vi "example_02_convert.vi"() -> ()   [LabVIEW 2015, in "lv-unit-conversion.lvlib"] (continued)
"underlying_def"="", "description"=""}, {"symbol"="gal[US]/lbm", "name"="US gallon per pound-mass", "dimension"="L3/M", "is_si_unit"=TRUE, "category"="derived", "base_unit"="m3/kg", "conversion_reference"="DERIVED", "is_exact"=TRUE, "a"=0.0, "b"=0.003785411784, "c"=0.45359237, "d"=0.0, "underlying_def"="", "description"=""}, {"symbol"="gal[US]/sack[94lbm]", "name"="US gallon per 94-pound-sack", "dimension"="L3/M", "is_si_unit"=TRUE, "category"="derived", "base_unit"="m3/kg", "conversion_reference"="DERIVED", "is_exact"=TRUE, "a"=0.0, "b"=0.003785411784, "c"=42.63768278, "d"=0.0, "underlying_def"="", "description"=""}, {"symbol"="gal[US]/ton[UK]", "name"="US gallon per UK ton-mass", "dimension"="L3/M", "is_si_unit"=TRUE, "category"="derived", "base_unit"="m3/kg", "conversion_reference"="DERIVED", "is_exact"=TRUE, "a"=0.0, "b"=0.003785411784, "c"=1016.0469088, "d"=0.0, "underlying_def"="", "description"=""}, {"symbol"="gal[US]/ton[US]", "name"="US gallon per US ton-mass", "dimension"="L3/M", "is_si_unit"=TRUE, "category"="derived", "base_unit"="m3/kg", "conversion_reference"="DERIVED", "is_exact"=TRUE, "a"=0.0, "b"=0.003785411784, "c"=907.18474, "d"=0.0, "underlying_def"="", "description"=""}, {"symbol"="L/kg", "name"="litre per kilogram", "dimension"="L3/M", "is_si_unit"=TRUE, "category"="derived", "base_unit"="m3/kg", "conversion_reference"="DERIVED", "is_exact"=TRUE, "a"=0.0, "b"=0.001, "c"=1.0, "d"=0.0, "underlying_def"="", "description"=""}, {"symbol"="L/t", "name"="litre per tonne", "dimension"="L3/M", "is_si_unit"=TRUE, "category"="derived", "base_unit"="m3/kg", "conversion_reference"="DERIVED", "is_exact"=TRUE, "a"=0.0, "b"=1e-06, "c"=1.0, "d"=0.0, "underlying_def"="", "description"=""}, {"symbol"="L/ton[UK]", "name"="litre per UK ton-mass", "dimension"="L3/M", "is_si_unit"=TRUE, "category"="derived", "base_unit"="m3/kg", "conversion_reference"="DERIVED", "is_exact"=TRUE, "a"=0.0, "b"=0.001, "c"=1016.0469088, "d"=0.0, "underlying_def"="", "description"=""}, {"symbol"="m3/g", "name"="cubic metre per gram", "dimension"="L3/M", "is_si_unit"=TRUE, "category"="derived", "base_unit"="m3/kg", "conversion_reference"="DERIVED", "is_exact"=TRUE, "a"=0.0, "b"=1000.0, "c"=1.0, "d"=0.0, "underlying_def"="", "description"=""}, {"symbol"="m3/t", "name"="cubic metre per tonne", "dimension"="L3/M", "is_si_unit"=TRUE, "category"="derived", "base_unit"="m3/kg", "conversion_reference"="DERIVED", "is_exact"=TRUE, "a"=0.0, "b"=0.001, "c"=1.0, "d"=0.0, "underlying_def"="", "description"=""}, {"symbol"="m3/ton[UK]", "name"="cubic metre per UK ton-mass", "dimension"="L3/M", "is_si_unit"=TRUE, "category"="derived", "base_unit"="m3/kg", "conversion_reference"="DERIVED", "is_exact"=TRUE, "a"=0.0, "b"=1.0, "c"=1016.0469088, "d"=0.0, "underlying_def"="", "description"=""}, {"symbol"="m3/ton[US]", "name"="cubic metre per US ton-mass", "dimension"="L3/M", "is_si_unit"=TRUE, "category"="derived", "base_unit"="m3/kg", "conversion_reference"="DERIVED", "is_exact"=TRUE, "a"=0.0, "b"=1.0, "c"=907.18474, "d"=0.0, "underlying_def"="", "description"=""}, {"symbol"="m3/mol", "name"="cubic metre per gram-mole", "dimension"="L3/N", "is_si_unit"=TRUE, "category"="derived", "base_unit"="", "conversion_reference"="", "is_exact"=FALSE, "a"=0.0, "b"=0.0, "c"=0.0, "d"=0.0, "underlying_def"="", "description"=""}, {"symbol"="dm3/kmol", "name"="cubic decimetre per kilogram-mole", "dimension"="L3/N", "is_si_unit"=TRUE, "category"="derived", "base_unit"="m3/mol", "conversion_reference"="DERIVED", "is_exact"=TRUE, "a"=0.0, "b"=1e-06, "c"=1.0, "d"=0.0, "underlying_def"="", "description"=""}, {"symbol"="ft3/lbmol", "name"="cubic foot per pound-mass-mole", "dimension"="L3/N", "is_si_unit"=TRUE, "category"="derived", "base_unit"="m3/mol", "conversion_reference"="DERIVED", "is_exact"=TRUE, "a"=0.0, "b"=0.028316846592, "c"=453.59237, "d"=0.0, "underlying_def"="", "description"=""}, {"symbol"="L/kmol", "name"="litre per kilogram-mole", "dimension"="L3/N", "is_si_unit"=TRUE, "category"="derived", "base_unit"="m3/mol", "conversion_reference"="DERIVED", "is_exact"=TRUE, "a"=0.0, "b"=1e-06, "c"=1.0, "d"=0.0, "underlying_def"="", "description"=""}, {"symbol"="L/mol", "name"="litre per gram-mole", "dimension"="L3/N", "is_si_unit"=TRUE, "category"="derived", "base_unit"="m3/mol", "conversion_reference"="DERIVED", "is_exact"=TRUE, "a"=0.0, "b"=0.001, "c"=1.0, "d"=0.0, "underlying_def"="", "description"=""}, {"symbol"="m3/kmol", "name"="cubic metre per kilogram-mole", "dimension"="L3/N", "is_si_unit"=TRUE, "category"="derived", "base_unit"="m3/mol", "conversion_reference"="DERIVED", "is_exact"=TRUE, "a"=0.0, "b"=0.001, "c"=1.0, "d"=0.0, "underlying_def"="", "description"=""}, {"symbol"="m3/s", "name"="cubic metre per second", "dimension"="L3/T", "is_si_unit"=TRUE, "category"="derived", "base_unit"="", "conversion_reference"="", "is_exact"=FALSE, "a"=0.0, "b"=0.0, "c"=0.0, "d"=0.0, "underlying_def"="", "description"=""}, {"symbol"="1/30 cm3/min", "name"="cubic centimetre per thirty minute", "dimension"="L3/T", "is_si_unit"=TRUE, "category"="derived", "base_unit"="m3/s", "conversion_reference"="DERIVED", "is_exact"=TRUE, "a"=0.0, "b"=1e-06, "c"=1800.0, "d"=0.0, "underlying_def"="", "description"=""}, {"symbol"="1000 bbl/d", "name"="thousand barrel per day", "dimension"="L3/T", "is_si_unit"=TRUE, "category"="derived", "base_unit"="m3/s", "conversion_reference"="DERIVED", "is_exact"=TRUE, "a"=0.0, "b"=158.987294928, "c"=86400.0, "d"=0.0, "underlying_def"="", "description"=""}, {"symbol"="1000 ft3/d", "name"="thousand cubic foot per day", "dimension"="L3/T", "is_si_unit"=TRUE, "category"="derived", "base_unit"="m3/s", "conversion_reference"="DERIVED", "is_exact"=TRUE, "a"=0.0, "b"=28.316846592, "c"=86400.0, "d"=0.0, "underlying_def"="", "description"=""}, {"symbol"="1000 m3/d", "name"="thousand cubic metre per day", "dimension"="L3/T", "is_si_unit"=TRUE, "category"="derived", "base_unit"="m3/s", "conversion_reference"="DERIVED", "is_exact"=TRUE, "a"=0.0, "b"=1000.0, "c"=86400.0, "d"=0.0, "underlying_def"="", "description"=""}, {"symbol"="1000 m3/h", "name"="thousand cubic metre per hour", "dimension"="L3/T", "is_si_unit"=TRUE, "category"="derived", "base_unit"="m3/s", "conversion_reference"="DERIVED", "is_exact"=TRUE, "a"=0.0, "b"=1000.0, "c"=3600.0, "d"=0.0, "underlying_def"="", "description"=""}, {"symbol"="1E6 bbl/d", "name"="million barrel per day", "dimension"="L3/T", "is_si_unit"=TRUE, "category"="derived", "base_unit"="m3/s", "conversion_reference"="DERIVED", "is_exact"=TRUE, "a"=0.0, "b"=158987.294928, "c"=86400.0, "d"=0.0, "underlying_def"="", "description"=""}, {"symbol"="1E6 ft3/d", "name"="million cubic foot per day", "dimension"="L3/T", "is_si_unit"=TRUE, "category"="derived", "base_unit"="m3/s", "conversion_reference"="DERIVED", "is_exact"=TRUE, "a"=0.0, "b"=28316.846592, "c"=86400.0, "d"=0.0, "underlying_def"="", "description"=""}, {"symbol"="1E6 m3/d", "name"="million cubic metre per day", "dimension"="L3/T", "is_si_unit"=TRUE, "category"="derived", "base_unit"="m3/s", "conversion_reference"="DERIVED", "is_exact"=TRUE, "a"=0.0, "b"=1000000.0, "c"=86400.0, "d"=0.0, "underlying_def"="", "description"=""}, {"symbol"="bbl/d", "name"="barrel per day", "dimension"="L3/T", "is_si_unit"=TRUE, "category"="derived", "base_unit"="m3/s", "conversion_reference"="DERIVED", "is_exact"=TRUE, "a"=0.0, "b"=0.158987294928, "c"=86400.0, "d"=0.0, "underlying_def"="", "description"=""}, {"symbol"="bbl/h", "name"="barrel per hour", "dimension"="L3/T", "is_si_unit"=TRUE, "category"="derived", "base_unit"="m3/s", "conversion_reference"="DERIVED", "is_exact"=TRUE, "a"=0.0, "b"=0.158987294928, "c"=3600.0, "d"=0.0, "underlying_def"="", "description"=""}, {"symbol"="bbl/min", "name"="barrel per minute", "dimension"="L3/T", "is_si_unit"=TRUE, "category"="derived", "base_unit"="m3/s", "conversion_reference"="DERIVED", "is_exact"=TRUE, "a"=0.0, "b"=0.158987294928, "c"=60.0, "d"=0.0, "underlying_def"="", "description"=""}, {"symbol"="cm3/h", "name"="cubic centimetre per hour", "dimension"="L3/T", "is_si_unit"=TRUE, "category"="derived", "base_unit"="m3/s", "conversion_reference"="DERIVED", "is_exact"=TRUE, "a"=0.0, "b"=1e-06, "c"=3600.0, "d"=0.0, "underlying_def"="", "description"=""}, {"symbol"="cm3/min", "name"="cubic centimetre per minute", "dimension"="L3/T", "is_si_unit"=TRUE, "category"="derived", "base_unit"="m3/s", "conversion_reference"="DERIVED", "is_exact"=TRUE, "a"=0.0, "b"=1e-06, "c"=60.0, "d"=0.0, "underlying_def"="", "description"=""}, {"symbol"="cm3/s", "name"="cubic centimetre per second", "dimension"="L3/T", "is_si_unit"=TRUE, "category"="derived", "base_unit"="m3/s", "conversion_reference"="DERIVED", "is_exact"=TRUE, "a"=0.0, "b"=1e-06, "c"=1.0, "d"=0.0, "underlying_def"="", "description"=""}, {"symbol"="dm3/s", "name"="cubic decimetre per second", "dimension"="L3/T", "is_si_unit"=TRUE, "category"="derived", "base_unit"="m3/s", "conversion_reference"="DERIVED", "is_exact"=TRUE, "a"=0.0, "b"=0.001, "c"=1.0, "d"=0.0, "underlying_def"="", "description"=""}, {"symbol"="ft3/d", "name"="cubic foot per day", "dimension"="L3/T", "is_si_unit"=TRUE, "category"="derived", "base_unit"="m3/s", "conversion_reference"="DERIVED", "is_exact"=TRUE, "a"=0.0, "b"=0.028316846592, "c"=86400.0, "d"=0.0, "underlying_def"="", "description"=""}, {"symbol"="ft3/h", "name"="cubic foot per hour", "dimension"="L3/T", "is_si_unit"=TRUE, "category"="derived", "base_unit"="m3/s", "conversion_reference"="DERIVED", "is_exact"=TRUE, "a"=0.0, "b"=0.028316846592, "c"=3600.0, "d"=0.0, "underlying_def"="", "description"=""}, {"symbol"="ft3/min", "name"="cubic foot per minute", "dimension"="L3/T", "is_si_unit"=TRUE, "category"="derived", "base_unit"="m3/s", "conversion_reference"="DERIVED", "is_exact"=TRUE, "a"=0.0, "b"=0.028316846592, "c"=60.0, "d"=0.0, "underlying_def"="", "description"=""}, {"symbol"="ft3/s", "name"="cubic foot per second", "dimension"="L3/T", "is_si_unit"=TRUE, "category"="derived", "base_unit"="m3/s", "conversion_reference"="DERIVED", "is_exact"=TRUE, "a"=0.0, "b"=0.028316846592, "c"=1.0, "d"=0.0, "underlying_def"="", "description"=""}, {"symbol"="gal[UK]/d", "name"="UK gallon per day", "dimension"="L3/T", "is_si_unit"=TRUE, "category"="derived", "base_unit"="m3/s", "conversion_reference"="DERIVED", "is_exact"=TRUE, "a"=0.0, "b"=0.00454609, "c"=86400.0, "d"=0.0, "underlying_def"="", "description"=""}, {"symbol"="gal[UK]/h", "name"="UK gallon per hour", "dimension"="L3/T", "is_si_unit"=TRUE, "category"="derived", "base_unit"="m3/s", "conversion_reference"="DERIVED", "is_exact"=TRUE, "a"=0.0, "b"=0.00454609, "c"=3600.0, "d"=0.0, "underlying_def"="", "description"=""}, {"symbol"="gal[UK]/min", "name"="UK gallon per minute", "dimension"="L3/T", "is_si_unit"=TRUE, "category"="derived", "base_unit"="m3/s", "conversion_reference"="DERIVED", "is_exact"=TRUE, "a"=0.0, "b"=0.00454609, "c"=60.0, "d"=0.0, "underlying_def"="", "description"=""}, {"symbol"="gal[US]/d", "name"="US gallon per day", "dimension"="L3/T", "is_si_unit"=TRUE, "category"="derived", "base_unit"="m3/s", "conversion_reference"="DERIVED", "is_exact"=TRUE, "a"=0.0, "b"=0.003785411784, "c"=86400.0, "d"=0.0, "underlying_def"="", "description"=""}, {"symbol"="gal[US]/h", "name"="US gallon per hour", "dimension"="L3/T", "is_si_unit"=TRUE, "category"="derived", "base_unit"="m3/s", "conversion_reference"="DERIVED", "is_exact"=TRUE, "a"=0.0, "b"=0.003785411784, "c"=3600.0, "d"=0.0, "underlying_def"="", "description"=""}, {"symbol"="gal[US]/min", "name"="US gallon per minute", "dimension"="L3/T", "is_si_unit"=TRUE, "category"="derived", "base_unit"="m3/s", "conversion_reference"="DERIVED", "is_exact"=TRUE, "a"=0.0, "b"=0.003785411784, "c"=60.0, "d"=0.0, "underlying_def"="", "description"=""}, {"symbol"="L/h", "name"="litre per hour", "dimension"="L3/T", "is_si_unit"=TRUE, "category"="derived", "base_unit"="m3/s", "conversion_reference"="DERIVED", "is_exact"=TRUE, "a"=0.0, "b"=0.001, "c"=3600.0, "d"=0.0, "underlying_def"="", "description"=""}, {"symbol"="L/min", "name"="litre per minute", "dimension"="L3/T", "is_si_unit"=TRUE, "category"="derived", "base_unit"="m3/s", "conversion_reference"="DERIVED", "is_exact"=TRUE, "a"=0.0, "b"=0.001, "c"=60.0, "d"=0.0, "underlying_def"="", "description"=""}, {"symbol"="L/s", "name"="litre per second", "dimension"="L3/T", "is_si_unit"=TRUE, "category"="derived", "base_unit"="m3/s", "conversion_reference"="DERIVED", "is_exact"=TRUE, "a"=0.0, "b"=0.001, "c"=1.0, "d"=0.0, "underlying_def"="", "description"=""}, {"symbol"="m3/d", "name"="cubic metre per day", "dimension"="L3/T", "is_si_unit"=TRUE, "category"="derived", "base_unit"="m3/s", "conversion_reference"="DERIVED", "is_exact"=TRUE, "a"=0.0, "b"=1.0, "c"=86400.0, "d"=0.0, "underlying_def"="", "description"=""}, {"symbol"="m3/h", "name"="cubic metre per hour", "dimension"="L3/T", "is_si_unit"=TRUE, "category"="derived", "base_unit"="m3/s", "conversion_reference"="DERIVED", "is_exact"=TRUE, "a"=0.0, "b"=1.0, "c"=3600.0, "d"=0.0, "underlying_def"="", "description"=""}, {"symbol"="m3/min", "name"="cubic metre per minute", "dimension"="L3/T", "is_si_unit"=TRUE, "category"="derived", "base_unit"="m3/s", "conversion_reference"="DERIVED", "is_exact"=TRUE, "a"=0.0, "b"=1.0, "c"=60.0, "d"=0.0, "underlying_def"="", "description"=""}, {"symbol"="m3/s2", "name"="cubic metre per second squared", "dimension"="L3/T2", "is_si_unit"=TRUE, "category"="derived", "base_unit"="", "conversion_reference"="", "is_exact"=FALSE, "a"=0.0, "b"=0.0, "c"=0.0, "d"=0.0, "underlying_def"="", "description"=""}, {"symbol"="bbl/d2", "name"="(barrel per day) per day", "dimension"="L3/T2", "is_si_unit"=TRUE, "category"="derived", "base_unit"="m3/s2", "conversion_reference"="DERIVED", "is_exact"=TRUE, "a"=0.0, "b"=0.158987294928, "c"=7464960000.0, "d"=0.0, "underlying_def"="", "description"=""}, {"symbol"="bbl/h2", "name"="(barrel per hour) per hour", "dimension"="L3/T2", "is_si_unit"=TRUE, "category"="derived", "base_unit"="m3/s2", "conversion_reference"="DERIVED", "is_exact"=TRUE, "a"=0.0, "b"=0.158987294928, "c"=12960000.0, "d"=0.0, "underlying_def"="", "description"=""}, {"symbol"="dm3/s2", "name"="(cubic decimetre per second) per second", "dimension"="L3/T2", "is_si_unit"=TRUE, "category"="derived", "base_unit"="m3/s2", "conversion_reference"="DERIVED", "is_exact"=TRUE, "a"=0.0, "b"=0.001, "c"=1.0, "d"=0.0, "underlying_def"="", "description"=""}, {"symbol"="ft3/d2", "name"="(cubic foot per day) per day", "dimension"="L3/T2", "is_si_unit"=TRUE, "category"="derived", "base_unit"="m3/s2", "conversion_reference"="DERIVED", "is_exact"=TRUE, "a"=0.0, "b"=0.028316846592, "c"=7464960000.0, "d"=0.0, "underlying_def"="", "description"=""}, {"symbol"="ft3/h2", "name"="(cubic foot per hour) per hour", "dimension"="L3/T2", "is_si_unit"=TRUE, "category"="derived", "base_unit"="m3/s2", "conversion_reference"="DERIVED", "is_exact"=TRUE, "a"=0.0, "b"=0.028316846592, "c"=12960000.0, "d"=0.0, "underlying_def"="", "description"=""}, {"symbol"="ft3/min2", "name"="(cubic foot per minute) per minute", "dimension"="L3/T2", "is_si_unit"=TRUE, "category"="derived", "base_unit"="m3/s2", "conversion_reference"="DERIVED", "is_exact"=TRUE, "a"=0.0, "b"=0.028316846592, "c"=3600.0, "d"=0.0, "underlying_def"="", "description"=""}, {"symbol"="ft3/s2", "name"="(cubic foot per second) per second", "dimension"="L3/T2", "is_si_unit"=TRUE, "category"="derived", "base_unit"="m3/s2", "conversion_reference"="DERIVED", "is_exact"=TRUE, "a"=0.0, "b"=0.028316846592, "c"=1.0, "d"=0.0, "underlying_def"="", "description"=""}, {"symbol"="gal[UK]/h2", "name"="(UK gallon per hour) per hour", "dimension"="L3/T2", "is_si_unit"=TRUE, "category"="derived", "base_unit"="m3/s2", "conversion_reference"="DERIVED", "is_exact"=TRUE, "a"=0.0, "b"=0.00454609, "c"=12960000.0, "d"=0.0, "underlying_def"="", "description"=""}, {"symbol"="gal[UK]/min2", "name"="(UK gallon per minute) per minute", "dimension"="L3/T2", "is_si_unit"=TRUE, "category"="derived", "base_unit"="m3/s2", "conversion_reference"="DERIVED", "is_exact"=TRUE, "a"=0.0, "b"=0.00454609, "c"=3600.0, "d"=0.0, "underlying_def"="", "description"=""}, {"symbol"="gal[US]/h2", "name"="(US gallon per hour) per hour", "dimension"="L3/T2", "is_si_unit"=TRUE, "category"="derived", "base_unit"="m3/s2", "conversion_reference"="DERIVED", "is_exact"=TRUE, "a"=0.0, "b"=0.003785411784, "c"=12960000.0, "d"=0.0, "underlying_def"="", "description"=""}, {"symbol"="gal[US]/min2", "name"="(US gallon per minute) per minute", "dimension"="L3/T2", "is_si_unit"=TRUE, "category"="derived", "base_unit"="m3/s2", "conversion_reference"="DERIVED", "is_exact"=TRUE, "a"=0.0, "b"=0.003785411784, "c"=3600.0, "d"=0.0, "underlying_def"="", "description"=""}, {"symbol"="L/s2", "name"="(litre per second) per second", "dimension"="L3/T2", "is_si_unit"=TRUE, "category"="derived", "base_unit"="m3/s2", "conversion_reference"="DERIVED", "is_exact"=TRUE, "a"=0.0, "b"=0.001, "c"=1.0, "d"=0.0, "underlying_def"="", "description"=""}, {"symbol"="m3/d2", "name"="(cubic metre per day) per day", "dimension"="L3/T2", "is_si_unit"=TRUE, "category"="derived", "base_unit"="m3/s2", "conversion_reference"="DERIVED", "is_exact"=TRUE, "a"=0.0, "b"=1.0, "c"=7464960000.0, "d"=0.0, "underlying_def"="", "description"=""}, {"symbol"="ohm.m", "name"="ohm metre", "dimension"="L3M/I2T3", "is_si_unit"=TRUE, "category"="derived", "base_unit"="", "conversion_reference"="", "is_exact"=FALSE, "a"=0.0, "b"=0.0, "c"=0.0, "d"=0.0, "underlying_def"="", "description"=""}, {"symbol"="kohm.m", "name"="kiloohm metre", "dimension"="L3M/I2T3", "is_si_unit"=TRUE, "category"="derived", "base_unit"="ohm.m", "conversion_reference"="DERIVED", "is_exact"=TRUE, "a"=0.0, "b"=1000.0, "c"=1.0, "d"=0.0, "underlying_def"="", "description"=""}, {"symbol"="nohm.mil2/ft", "name"="nanoohm square mil per foot", "dimension"="L3M/I2T3", "is_si_unit"=TRUE, "category"="derived", "base_unit"="ohm.m", "conversion_reference"="DERIVED", "is_exact"=TRUE, "a"=0.0, "b"=6.4516e-19, "c"=0.3048, "d"=0.0, "underlying_def"="", "description"=""}, {"symbol"="nohm.mm2/m", "name"="nanoohm square milimetre per metre", "dimension"="L3M/I2T3", "is_si_unit"=TRUE, "category"="derived", "base_unit"="ohm.m", "conversion_reference"="DERIVED", "is_exact"=TRUE, "a"=0.0, "b"=1e-15, "c"=1.0, "d"=0.0, "underlying_def"="", "description"=""}, {"symbol"="ohm.cm", "name"="ohm centimetre", "dimension"="L3M/I2T3", "is_si_unit"=TRUE, "category"="derived", "base_unit"="ohm.m", "conversion_reference"="DERIVED", "is_exact"=TRUE, "a"=0.0, "b"=0.01, "c"=1.0, "d"=0.0, "underlying_def"="", "description"=""}, {"symbol"="ohm.m2/m", "name"="ohm square metre per metre", "dimension"="L3M/I2T3", "is_si_unit"=TRUE, "category"="derived", "base_unit"="ohm.m", "conversion_reference"="DERIVED", "is_exact"=TRUE, "a"=0.0, "b"=1.0, "c"=1.0, "d"=0.0, "underlying_def"="", "description"=""}, {"symbol"="Wb.m", "name"="weber metre", "dimension"="L3M/IT2", "is_si_unit"=TRUE, "category"="derived", "base_unit"="", "conversion_reference"="", "is_exact"=FALSE, "a"=0.0, "b"=0.0, "c"=0.0, "d"=0.0, "underlying_def"="", "description"=""}, {"symbol"="N.m2", "name"="newton square metre", "dimension"="L3M/T2", "is_si_unit"=TRUE, "category"="derived", "base_unit"="", "conversion_reference"="", "is_exact"=FALSE, "a"=0.0, "b"=0.0, "c"=0.0, "d"=0.0, "underlying_def"="", "description"=""}, {"symbol"="dyne.cm2", "name"="dyne square centimetre", "dimension"="L3M/T2", "is_si_unit"=TRUE, "category"="derived", "base_unit"="N.m2", "conversion_reference"="DERIVED", "is_exact"=TRUE, "a"=0.0, "b"=1e-09, "c"=1.0, "d"=0.0, "underlying_def"="", "description"=""}, {"symbol"="kgf.m2", "name"="thousand gram-force square metre", "dimension"="L3M/T2", "is_si_unit"=TRUE, "category"="derived", "base_unit"="N.m2", "conversion_reference"="DERIVED", "is_exact"=TRUE, "a"=0.0, "b"=9.80665, "c"=1.0, "d"=0.0, "underlying_def"="", "description"=""}, {"symbol"="kN.m2", "name"="kilonewton square metre", "dimension"="L3M/T2", "is_si_unit"=TRUE, "category"="derived", "base_unit"="N.m2", "conversion_reference"="DERIVED", "is_exact"=TRUE, "a"=0.0, "b"=1000.0, "c"=1.0, "d"=0.0, "underlying_def"="", "description"=""}, {"symbol"="lbf.in2", "name"="pound-force square inch", "dimension"="L3M/T2", "is_si_unit"=TRUE, "category"="derived", "base_unit"="N.m2", "conversion_reference"="DERIVED", "is_exact"=TRUE, "a"=0.0, "b"=0.002869814657301464, "c"=1.0, "d"=0.0, "underlying_def"="", "description"=""}, {"symbol"="mN.m2", "name"="millinewton square metre", "dimension"="L3M/T2", "is_si_unit"=TRUE, "category"="derived", "base_unit"="N.m2", "conversion_reference"="DERIVED", "is_exact"=TRUE, "a"=0.0, "b"=0.001, "c"=1.0, "d"=0.0, "underlying_def"="", "description"=""}, {"symbol"="pdl.cm2", "name"="poundal square centimetre", "dimension"="L3M/T2", "is_si_unit"=TRUE, "category"="derived", "base_unit"="N.m2", "conversion_reference"="DERIVED", "is_exact"=TRUE, "a"=0.0, "b"=1.38254954376e-05, "c"=1.0, "d"=0.0, "underlying_def"="", "description"=""}, {"symbol"="tonf[UK].ft2", "name"="UK ton-force square foot", "dimension"="L3M/T2", "is_si_unit"=TRUE, "category"="derived", "base_unit"="N.m2", "conversion_reference"="DERIVED", "is_exact"=TRUE, "a"=0.0, "b"=925.6874158591603, "c"=1.0, "d"=0.0, "underlying_def"="", "description"=""}, {"symbol"="tonf[US].ft2", "name"="US ton-force square foot", "dimension"="L3M/T2", "is_si_unit"=TRUE, "category"="derived", "base_unit"="N.m2", "conversion_reference"="DERIVED", "is_exact"=TRUE, "a"=0.0, "b"=826.5066213028217, "c"=1.0, "d"=0.0, "underlying_def"="", "description"=""}, {"symbol"="m2/(Pa.s)", "name"="square metre per pascal second", "dimension"="L3T/M", "is_si_unit"=TRUE, "category"="derived", "base_unit"="", "conversion_reference"="", "is_exact"=FALSE, "a"=0.0, "b"=0.0, "c"=0.0, "d"=0.0, "underlying_def"="", "description"=""}, {"symbol"="TD[API]/(Pa.s)", "name"="teradarcy-API per pascal second", "dimension"="L3T/M", "is_si_unit"=TRUE, "category"="derived", "base_unit"="", "conversion_reference"="", "is_exact"=FALSE, "a"=0.0, "b"=0.0, "c"=0.0, "d"=0.0, "underlying_def"="m2/(Pa.s)", "description"=""}, {"symbol"="bbl/(ft.psi.d)", "name"="barrel per day foot psi", "dimension"="L3T/M", "is_si_unit"=TRUE, "category"="derived", "base_unit"="m2/(Pa.s)", "conversion_reference"="DERIVED", "is_exact"=TRUE, "a"=0.0, "b"=0.00010257224319574849, "c"=117142.67073583299, "d"=0.0, "underlying_def"="", "description"=""}, {"symbol"="ft3/(ft.psi.d)", "name"="cubic foot per day foot psi", "dimension"="L3T/M", "is_si_unit"=TRUE, "category"="derived", "base_unit"="m2/(Pa.s)", "conversion_reference"="DERIVED", "is_exact"=TRUE, "a"=0.0, "b"=5.99373252864e-05, "c"=384326.3475585072, "d"=0.0, "underlying_def"="", "description"=""}, {"symbol"="m2/(kPa.d)", "name"="square metre per kilopascal day", "dimension"="L3T/M", "is_si_unit"=TRUE, "category"="derived", "base_unit"="m2/(Pa.s)", "conversion_reference"="DERIVED", "is_exact"=TRUE, "a"=0.0, "b"=1.0, "c"=86400000.0, "d"=0.0, "underlying_def"="", "description"=""}, {"symbol"="D/(Pa.s)", "name"="darcy per pascal second", "dimension"="L3T/M", "is_si_unit"=TRUE, "category"="derived", "base_unit"="TD[API]/(Pa.s)", "conversion_reference"="DERIVED", "is_exact"=TRUE, "a"=0.0, "b"=1e-12, "c"=1.01325, "d"=0.0, "underlying_def"="", "description"=""}, {"symbol"="D/cP", "name"="darcy per centipoise", "dimension"="L3T/M", "is_si_unit"=TRUE, "category"="derived", "base_unit"="TD[API]/(Pa.s)", "conversion_reference"="DERIVED", "is_exact"=TRUE, "a"=0.0, "b"=1e-09, "c"=1.01325, "d"=0.0, "underlying_def"="", "description"=""}, {"symbol"="mD.ft2/(lbf.s)", "name"="millidarcy square foot per pound-force second", "dimension"="L3T/M", "is_si_unit"=TRUE, "category"="derived", "base_unit"="TD[API]/(Pa.s)", "conversion_reference"="DERIVED", "is_exact"=TRUE, "a"=0.0, "b"=9.290304e-17, "c"=4.507160551662702, "d"=0.0, "underlying_def"="", "description"=""}, {"symbol"="mD.in2/(lbf.s)", "name"="millidarcy square inch per pound-force second", "dimension"="L3T/M", "is_si_unit"=TRUE, "category"="derived", "base_unit"="TD[API]/(Pa.s)", "conversion_reference"="DERIVED", "is_exact"=TRUE, "a"=0.0, "b"=6.4516e-19, "c"=4.507160551662702, "d"=0.0, "underlying_def"="", "description"=""}, {"symbol"="mD/(Pa.s)", "name"="millidarcy per pascal second", "dimension"="L3T/M", "is_si_unit"=TRUE, "category"="derived", "base_unit"="TD[API]/(Pa.s)", "conversion_reference"="DERIVED", "is_exact"=TRUE, "a"=0.0, "b"=1e-15, "c"=1.01325, "d"=0.0, "underlying_def"="", "description"=""}, {"symbol"="mD/cP", "name"="millidarcy per centipoise", "dimension"="L3T/M", "is_si_unit"=TRUE, "category"="derived", "base_unit"="TD[API]/(Pa.s)", "conversion_reference"="DERIVED", "is_exact"=TRUE, "a"=0.0, "b"=1e-12, "c"=1.01325, "d"=0.0, "underlying_def"="", "description"=""}, {"symbol"="cm4", "name"="centimetre to the fourth power", "dimension"="L4", "is_si_unit"=TRUE, "category"="derived", "base_unit"="m4", "conversion_reference"="DERIVED", "is_exact"=TRUE, "a"=0.0, "b"=1e-08, "c"=1.0, "d"=0.0, "underlying_def"="", "description"=""}, {"symbol"="m4", "name"="metre to the fourth power", "dimension"="L4", "is_si_unit"=TRUE, "category"="derived", "base_unit"="", "conversion_reference"="", "is_exact"=FALSE, "a"=0.0, "b"=0.0, "c"=0.0, "d"=0.0, "underlying_def"="", "description"=""}, {"symbol"="in4", "name"="inch to the fourth power", "dimension"="L4", "is_si_unit"=TRUE, "category"="derived", "base_unit"="m4", "conversion_reference"="DERIVED", "is_exact"=TRUE, "a"=0.0, "b"=4.162314256e-07, "c"=1.0, "d"=0.0, "underlying_def"="", "description"=""}, {"symbol"="m4/s", "name"="metre to the fourth power per second", "dimension"="L4/T", "is_si_unit"=TRUE, "category"="derived", "base_unit"="", "conversion_reference"="", "is_exact"=FALSE, "a"=0.0, "b"=0.0, "c"=0.0, "d"=0.0, "underlying_def"="", "description"=""}, {"symbol"="1000 bbl.ft/d", "name"="thousand barrel foot per day", "dimension"="L4/T", "is_si_unit"=TRUE, "category"="derived", "base_unit"="m4/s", "conversion_reference"="DERIVED", "is_exact"=TRUE, "a"=0.0, "b"=48.4593274940544, "c"=86400.0, "d"=0.0, "underlying_def"="", "description"=""}, {"symbol"="1000 m4/d", "name"="thousand (cubic metre per day) metre", "dimension"="L4/T", "is_si_unit"=TRUE, "category"="derived", "base_unit"="m4/s", "conversion_reference"="DERIVED", "is_exact"=TRUE, "a"=0.0, "b"=1000.0, "c"=86400.0, "d"=0.0, "underlying_def"="", "description"=""}, {"symbol"="m3/(Pa.s)", "name"="cubic metre per pascal second", "dimension"="L4T/M", "is_si_unit"=TRUE, "category"="derived", "base_unit"="", "conversion_reference"="", "is_exact"=FALSE, "a"=0.0, "b"=0.0, "c"=0.0, "d"=0.0, "underlying_def"="", "description"=""}, {"symbol"="1000 ft3/(psi.d)", "name"="(thousand cubic foot per day) per psi", "dimension"="L4T/M", "is_si_unit"=TRUE, "category"="derived", "base_unit"="m3/(Pa.s)", "conversion_reference"="DERIVED", "is_exact"=TRUE, "a"=0.0, "b"=0.01826889674729472, "c"=384326.3475585072, "d"=0.0, "underlying_def"="", "description"=""}, {"symbol"="bbl/(kPa.d)", "name"="(barrel per day) per kilopascal", "dimension"="L4T/M", "is_si_unit"=TRUE, "category"="derived", "base_unit"="m3/(Pa.s)", "conversion_reference"="DERIVED", "is_exact"=TRUE, "a"=0.0, "b"=0.158987294928, "c"=86400000.0, "d"=0.0, "underlying_def"="", "description"=""}, {"symbol"="bbl/(psi.d)", "name"="(barrel per day) per psi", "dimension"="L4T/M", "is_si_unit"=TRUE, "category"="derived", "base_unit"="m3/(Pa.s)", "conversion_reference"="DERIVED", "is_exact"=TRUE, "a"=0.0, "b"=0.00010257224319574849, "c"=384326.3475585072, "d"=0.0, "underlying_def"="", "description"=""}, {"symbol"="L/(bar.min)", "name"="(litre per minute) per bar", "dimension"="L4T/M", "is_si_unit"=TRUE, "category"="derived", "base_unit"="m3/(Pa.s)", "conversion_reference"="DERIVED", "is_exact"=TRUE, "a"=0.0, "b"=0.001, "c"=6000000.0, "d"=0.0, "underlying_def"="", "description"=""}, {"symbol"="m3/(bar.d)", "name"="(cubic metre per day) per bar", "dimension"="L4T/M", "is_si_unit"=TRUE, "category"="derived", "base_unit"="m3/(Pa.s)", "conversion_reference"="DERIVED", "is_exact"=TRUE, "a"=0.0, "b"=1.0, "c"=8640000000.0, "d"=0.0, "underlying_def"="", "description"=""}, {"symbol"="m3/(bar.h)", "name"="(cubic metre per hour) per bar", "dimension"="L4T/M", "is_si_unit"=TRUE, "category"="derived", "base_unit"="m3/(Pa.s)", "conversion_reference"="DERIVED", "is_exact"=TRUE, "a"=0.0, "b"=1.0, "c"=360000000.0, "d"=0.0, "underlying_def"="", "description"=""}, {"symbol"="m3/(bar.min)", "name"="(cubic metre per minute) per bar", "dimension"="L4T/M", "is_si_unit"=TRUE, "category"="derived", "base_unit"="m3/(Pa.s)", "conversion_reference"="DERIVED", "is_exact"=TRUE, "a"=0.0, "b"=1.0, "c"=6000000.0, "d"=0.0, "underlying_def"="", "description"=""}, {"symbol"="m3/(kPa.d)", "name"="(cubic metre per day) per kilopascal", "dimension"="L4T/M", "is_si_unit"=TRUE, "category"="derived", "base_unit"="m3/(Pa.s)", "conversion_reference"="DERIVED", "is_exact"=TRUE, "a"=0.0, "b"=1.0, "c"=86400000.0, "d"=0.0, "underlying_def"="", "description"=""}, {"symbol"="m3/(kPa.h)", "name"="(cubic metre per hour) per kilopascal", "dimension"="L4T/M", "is_si_unit"=TRUE, "category"="derived", "base_unit"="m3/(Pa.s)", "conversion_reference"="DERIVED", "is_exact"=TRUE, "a"=0.0, "b"=1.0, "c"=3600000.0, "d"=0.0, "underlying_def"="", "description"=""}, {"symbol"="m3/(psi.d)", "name"="(cubic metre per day) per psi", "dimension"="L4T/M", "is_si_unit"=TRUE, "category"="derived", "base_unit"="m3/(Pa.s)", "conversion_reference"="DERIVED", "is_exact"=TRUE, "a"=0.0, "b"=0.00064516, "c"=384326.3475585072, "d"=0.0, "underlying_def"="", "description"=""}, {"symbol"="m3/Pa", "name"="cubic metre per Pascal", "dimension"="L4T2/M", "is_si_unit"=TRUE, "category"="derived", "base_unit"="", "conversion_reference"="", "is_exact"=FALSE, "a"=0.0, "b"=0.0, "c"=0.0, "d"=0.0, "underlying_def"="", "description"=""}, {"symbol"="bbl/psi", "name"="barrel per psi", "dimension"="L4T2/M", "is_si_unit"=TRUE, "category"="derived", "base_unit"="m3/Pa", "conversion_reference"="DERIVED", "is_exact"=TRUE, "a"=0.0, "b"=0.00010257224319574849, "c"=4.4482216152605, "d"=0.0, "underlying_def"="", "description"=""}, {"symbol"="m3/kPa", "name"="cubic metre per kilopascal", "dimension"="L4T2/M", "is_si_unit"=TRUE, "category"="derived", "base_unit"="m3/Pa", "conversion_reference"="DERIVED", "is_exact"=TRUE, "a"=0.0, "b"=0.001, "c"=1.0, "d"=0.0, "underlying_def"="", "description"=""}, {"symbol"="kg.m", "name"="kilogram metre", "dimension"="LM", "is_si_unit"=TRUE, "category"="derived", "base_unit"="", "conversion_reference"="", "is_exact"=FALSE, "a"=0.0, "b"=0.0, "c"=0.0, "d"=0.0, "underlying_def"="", "description"=""}, {"symbol"="lbm.ft", "name"="pound-mass foot", "dimension"="LM", "is_si_unit"=TRUE, "category"="derived", "base_unit"="kg.m", "conversion_reference"="DERIVED", "is_exact"=TRUE, "a"=0.0, "b"=0.138254954376, "c"=1.0, "d"=0.0, "underlying_def"="", "description"=""}, {"symbol"="J.m/(s.m2.deltaK)", "name"="joule metre per second square metre delta kelvin", "dimension"="LM/DT3", "is_si_unit"=TRUE, "category"="derived", "base_unit"="", "conversion_reference"="", "is_exact"=FALSE, "a"=0.0, "b"=0.0, "c"=0.0, "d"=0.0, "underlying_def"="W/(m.deltaK)", "description"=""}, {"symbol"="W/(m.deltaK)", "name"="watt per metre delta kelvin", "dimension"="LM/DT3", "is_si_unit"=TRUE, "category"="derived", "base_unit"="", "conversion_reference"="", "is_exact"=FALSE, "a"=0.0, "b"=0.0, "c"=0.0, "d"=0.0, "underlying_def"="", "description"=""}, {"symbol"="Btu[IT].in/(h.ft2.deltaF)", "name"="BTU per (hour square foot delta Fahrenheit per inch)", "dimension"="LM/DT3", "is_si_unit"=TRUE, "category"="derived", "base_unit"="J.m/(s.m2.deltaK)", "conversion_reference"="DERIVED", "is_exact"=TRUE, "a"=0.0, "b"=241.185767908932, "c"=1672.25472, "d"=0.0, "underlying_def"="", "description"=""}, {"symbol"="kJ.m/(h.m2.deltaK)", "name"="kilojoule metre per hour square metre delta kelvin", "dimension"="LM/DT3", "is_si_unit"=TRUE, "category"="derived", "base_unit"="J.m/(s.m2.deltaK)", "conversion_reference"="DERIVED", "is_exact"=TRUE, "a"=0.0, "b"=1.0, "c"=3.6, "d"=0.0, "underlying_def"="", "description"=""}, {"symbol"="Btu[IT]/(h.ft.deltaF)", "name"="BTU per hour foot delta Fahrenheit", "dimension"="LM/DT3", "is_si_unit"=TRUE, "category"="derived", "base_unit"="W/(m.deltaK)", "conversion_reference"="DERIVED", "is_exact"=TRUE, "a"=0.0, "b"=9495.50267358, "c"=5486.4, "d"=0.0, "underlying_def"="", "description"=""}, {"symbol"="cal[th]/(h.cm.deltaC)", "name"="calorie per hour centimetre delta Celsius", "dimension"="LM/DT3", "is_si_unit"=TRUE, "category"="derived", "base_unit"="W/(m.deltaK)", "conversion_reference"="DERIVED", "is_exact"=TRUE, "a"=0.0, "b"=4.184, "c"=36.0, "d"=0.0, "underlying_def"="", "description"=""}, {"symbol"="cal[th]/(s.cm.deltaC)", "name"="calorie per second centimetre delta Celsius", "dimension"="LM/DT3", "is_si_unit"=TRUE, "category"="derived", "base_unit"="W/(m.deltaK)", "conversion_reference"="DERIVED", "is_exact"=TRUE, "a"=0.0, "b"=418.4, "c"=1.0, "d"=0.0, "underlying_def"="", "description"=""}, {"symbol"="kcal[th]/(h.m.deltaC)", "name"="thousand calorie per hour metre delta Celsius", "dimension"="LM/DT3", "is_si_unit"=TRUE, "category"="derived", "base_unit"="W/(m.deltaK)", "conversion_reference"="DERIVED", "is_exact"=TRUE, "a"=0.0, "b"=4184.0, "c"=3600.0, "d"=0.0, "underlying_def"="", "description"=""}, {"symbol"="uH/m", "name"="microhenry per metre", "dimension"="LM/I2T2", "is_si_unit"=TRUE, "category"="derived", "base_unit"="H/m", "conversion_reference"="DERIVED", "is_exact"=TRUE, "a"=0.0, "b"=1e-06, "c"=1.0, "d"=0.0, "underlying_def"="", "description"=""}, {"symbol"="H/m", "name"="henry per metre", "dimension"="LM/I2T2", "is_si_unit"=TRUE, "category"="derived", "base_unit"="", "conversion_reference"="", "is_exact"=FALSE, "a"=0.0, "b"=0.0, "c"=0.0, "d"=0.0, "underlying_def"="", "description"=""}, {"symbol"="ohm/m", "name"="ohm per metre", "dimension"="LM/I2T3", "is_si_unit"=TRUE, "category"="derived", "base_unit"="", "conversion_reference"="", "is_exact"=FALSE, "a"=0.0, "b"=0.0, "c"=0.0, "d"=0.0, "underlying_def"="", "description"=""}, {"symbol"="uohm/ft", "name"="microhm per foot", "dimension"="LM/I2T3", "is_si_unit"=TRUE, "category"="derived", "base_unit"="ohm/m", "conversion_reference"="DERIVED", "is_exact"=TRUE, "a"=0.0, "b"=1e-06, "c"=0.3048, "d"=0.0, "underlying_def"="", "description"=""}, {"symbol"="uohm/m", "name"="microhm per metre", "dimension"="LM/I2T3", "is_si_unit"=TRUE, "category"="derived", "base_unit"="ohm/m", "conversion_reference"="DERIVED", "is_exact"=TRUE, "a"=0.0, "b"=1e-06, "c"=1.0, "d"=0.0, "underlying_def"="", "description"=""}, {"symbol"="Wb/m", "name"="weber per metre", "dimension"="LM/IT2", "is_si_unit"=TRUE, "category"="derived", "base_unit"="", "conversion_reference"="", "is_exact"=FALSE, "a"=0.0, "b"=0.0, "c"=0.0, "d"=0.0, "underlying_def"="", "description"=""}, {"symbol"="Wb/mm", "name"="weber per millimetre", "dimension"="LM/IT2", "is_si_unit"=TRUE, "category"="derived", "base_unit"="Wb/m", "conversion_reference"="DERIVED", "is_exact"=TRUE, "a"=0.0, "b"=1000.0, "c"=1.0, "d"=0.0, "underlying_def"="", "description"=""}, {"symbol"="V/m", "name"="volt per metre", "dimension"="LM/IT3", "is_si_unit"=TRUE, "category"="derived", "base_unit"="", "conversion_reference"="", "is_exact"=FALSE, "a"=0.0, "b"=0.0, "c"=0.0, "d"=0.0, "underlying_def"="", "description"=""}, {"symbol"="mV/ft", "name"="millivolt per foot", "dimension"="LM/IT3", "is_si_unit"=TRUE, "category"="derived", "base_unit"="V/m", "conversion_reference"="DERIVED", "is_exact"=TRUE, "a"=0.0, "b"=0.001, "c"=0.3048, "d"=0.0, "underlying_def"="", "description"=""}, {"symbol"="mV/m", "name"="millivolt per metre", "dimension"="LM/IT3", "is_si_unit"=TRUE, "category"="derived", "base_unit"="V/m", "conversion_reference"="DERIVED", "is_exact"=TRUE, "a"=0.0, "b"=0.001, "c"=1.0, "d"=0.0, "underlying_def"="", "description"=""}, {"symbol"="uV/ft", "name"="microvolt per foot", "dimension"="LM/IT3", "is_si_unit"=TRUE, "category"="derived", "base_unit"="V/m", "conversion_reference"="DERIVED", "is_exact"=TRUE, "a"=0.0, "b"=1e-06, "c"=0.3048, "d"=0.0, "underlying_def"="", "description"=""}, {"symbol"="uV/m", "name"="microvolt per metre", "dimension"="LM/IT3", "is_si_unit"=TRUE, "category"="derived", "base_unit"="V/m", "conversion_reference"="DERIVED", "is_exact"=TRUE, "a"=0.0, "b"=1e-06, "c"=1.0, "d"=0.0, "underlying_def"="", "description"=""}, {"symbol"="kg.m/s", "name"="kilogram metre per second", "dimension"="LM/T", "is_si_unit"=TRUE, "category"="derived", "base_unit"="", "conversion_reference"="", "is_exact"=FALSE, "a"=0.0, "b"=0.0, "c"=0.0, "d"=0.0, "underlying_def"="", "description"=""}, {"symbol"="lbm.ft/s", "name"="foot pound-mass per second", "dimension"="LM/T", "is_si_unit"=TRUE, "category"="derived", "base_unit"="kg.m/s", "conversion_reference"="DERIVED", "is_exact"=TRUE, "a"=0.0, "b"=0.138254954376, "c"=1.0, "d"=0.0, "underlying_def"="", "description"=""}, {"symbol"="N", "name"="newton", "dimension"="LM/T2", "is_si_unit"=TRUE, "category"="atom-special", "base_unit"="", "conversion_reference"="", "is_exact"=FALSE, "a"=0.0, "b"=0.0, "c"=0.0, "d"=0.0, "underlying_def"="m.kg/s2", "description"="That force which, when applied to a body having a mass of 1 kg, gives it an acceleration of 1 m/s2."}, {"symbol"="dyne", "name"="dyne", "dimension"="LM/T2", "is_si_unit"=TRUE, "category"="atom", "base_unit"="N", "conversion_reference"="NIST-SI", "is_exact"=TRUE, "a"=0.0, "b"=1e-05, "c"=1.0, "d"=0.0, "underlying_def"="(g.cm)/s2", "description"="A unit of force in the centimetre-gram-second system of physical units, equal to the force that \n\t\t\t\twould give a free mass of one gram an acceleration of one centimetre per second per second.\n\t\t\t"}, {"symbol"="gf", "name"="gram-force", "dimension"="LM/T2", "is_si_unit"=TRUE, "category"="atom", "base_unit"="N", "conversion_reference"="NIST-SI", "is_exact"=TRUE, "a"=0.0, "b"=0.00980665, "c"=1.0, "d"=0.0, "underlying_def"="g.gn", "description"="The gram-force is equal to a mass of one gram multiplied by the standard acceleration due to gravity \n\t\t\t\ton Earth, which is defined as exactly 9.80665 meter per second squared.\n\t\t\t"}, {"symbol"="lbf", "name"="pound-force", "dimension"="LM/T2", "is_si_unit"=TRUE, "category"="atom", "base_unit"="N", "conversion_reference"="NIST-SI", "is_exact"=TRUE, "a"=0.0, "b"=4.4482216152605, "c"=1.0, "d"=0.0, "underlying_def"="lbm.gn", "description"="The pound-force is equal to the gravitational force exerted on a mass of one avoirdupois pound on \n\t\t\t\tthe surface of Earth. \n\t\t\t\tThe exact conversion factor is 4.448 221 615 260 5 E+00 since the standard value of the acceleration \n\t\t\t\tdue to gravity, gn = 9.806 65 m/s2 exactly, is used to define the kilogram-force: 1 kgf = 9.806 65 \n\t\t\t\tE+00 N exactly.\n\t\t\t"}, {"symbol"="ozf", "name"="ounce-force", "dimension"="LM/T2", "is_si_unit"=TRUE, "category"="atom", "base_unit"="N", "conversion_reference"="DEFINITION", "is_exact"=TRUE, "a"=0.0, "b"=4.4482216152605, "c"=16.0, "d"=0.0, "underlying_def"="1/16 lbf", "description"="ounce (avoirdupois)-force"}, {"symbol"="pdl", "name"="poundal", "dimension"="LM/T2", "is_si_unit"=TRUE, "category"="atom", "base_unit"="N", "conversion_reference"="DEFINITION", "is_exact"=TRUE, "a"=0.0, "b"=0.138254954376, "c"=1.0, "d"=0.0, "underlying_def"="(lbm.ft)/s2", "description"="A unit of force equal to the force that would give a free mass of one pound an acceleration of one \n\t\t\t\tfoot per second per second [i.e., \"(lbm.ft)/s2\"]. \n\t\t\t\tTherefore, 1 pdl = 0.138254954376 N exactly. \n\t\t\t\tFrom merriam-webster.com.\n\t\t\t"}, {"symbol"="tonf[UK]", "name"="UK ton-force", "dimension"="LM/T2", "is_si_unit"=TRUE, "category"="atom", "base_unit"="N", "conversion_reference"="UK-1995", "is_exact"=TRUE, "a"=0.0, "b"=9964.01641818352, "c"=1.0, "d"=0.0, "underlying_def"="2240 lbf", "description"="United 
